vi "Find Pupil.vi"(11 "error in":errorcluster) -> (4 "Pupil Data":T1, 15 "error out":errorcluster)   [LabVIEW 2014]
uses:
  <vilib>/vision/NI_Vision_Development_Module.lvlib
panel:
  out "Image Out":T2(plugin-control)
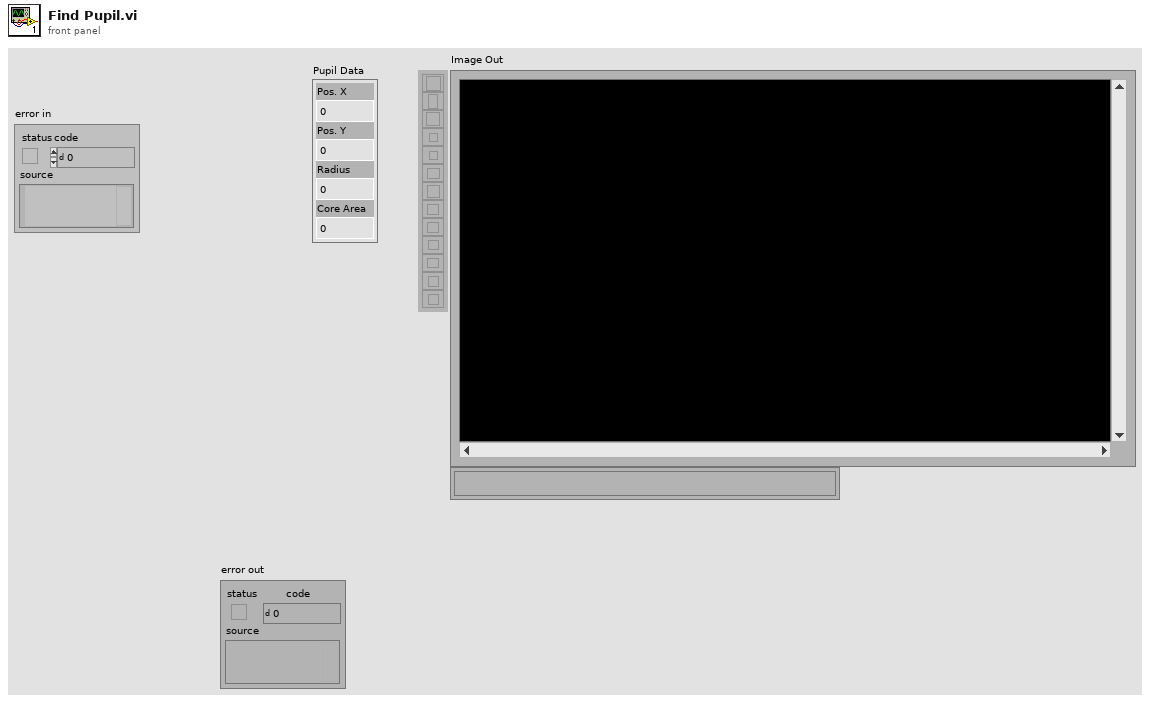
[diagram p1: front panel]
types:
  T1 = cluster{"Pos. X":i32, "Pos. Y":i32, "Radius":i32, "Core Area":i32}
  T2 = typedef "IMAQ Image.ctl" = refnum<image>
  T3 = cluster{"Left":i32, "Top":i32, "Right":i32, "Bottom":i32}
  T4 = typedef "Image Type" = u32
  T5 = cluster{"Pos. X":i32, "Pos. Y":i32, "Radius":i32, "Core Area":i32}[]
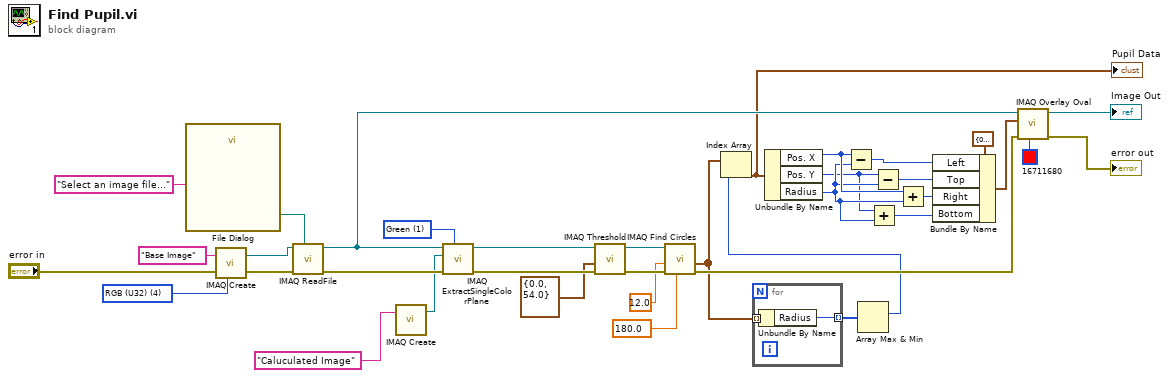
[diagram p0: block diagram]
diagram:
  w29 = 1 items=["Red", "Green", "Blue", "Hue", "Saturation", "Luminance", "Value", "Intensity"] ("Color Plane")
  w30 = T4 4 items=["Grayscale (U8)", "Grayscale (I16)", "Grayscale (SGL)", "Complex (CSG)", "RGB (U32)", "HSL (U32)", "RGB (U64)", "Grayscale (U16)"] ("Image Type")
  n1 = call "File Dialog"("prompt"="Select an image file...") -> ("selected path"=w31:path)  [unwired: 6 in, 8 out]
  n2 = call "IMAQ Create"("Image Name"="Base Image", "Image Type"=w30, "error in (no error)"="error in") -> ("New Image"=w35:T2, "error out"=w34:errorcluster)  [unwired: 1 in, 1 out]
  n3 = call "IMAQ ReadFile"("File Path"=w31, "error in (no error)"=w34, "Image"=w35) -> ("error out"=w36:errorcluster, "Image Out"=w19:T2)  [unwired: 2 in, 5 out]
  n4 = call "IMAQ Create"("Image Name"="Caluculated Image") -> ("New Image"=w20:T2)  [unwired: 3 in, 2 out]
  n5 = call "IMAQ ExtractSingleColorPlane"("Color Plane"=w29, "error in (no error)"=w36, "Image Dst"=w20, "Image Src"=w19) -> ("error out"=w28:errorcluster, "Image Dst Out"=w26:T2)  [unwired: 6 out]
  n6 = call "IMAQ Threshold"("error in (no error)"=w28, "Range"=cluster{"Lower value":sgl, "Upper value":sgl} {"Lower value"=0.0, "Upper value"=54.0}, "Image Src"=w26) -> ("error out"=w21:errorcluster, "Image Dst Out"=w24:T2)  [unwired: 3 in, 4 out]
  n7 = call "IMAQ Find Circles"("Max Radius"=sgl 180.0, "error in (no error)"=w21, "Min Radius"=sgl 12.0, "Image Src"=w24) -> ("error out"=w6:errorcluster, "Circles Data"=w4:T5)  [unwired: 1 in, 5 out]
  n8 = for {
    tunnel: w4 -> [w38] mode=indexing
    tunnel: [w37] -> w3 mode=indexing
    n9 = Unbundle By Name(w38) -> ("Radius"=w37:i32)
  }
  n10 = Array Max & Min(array=w3) -> (max index (indices)=w2:i32)  [unwired: 3 out]
  n11 = Index Array(array=w4, index=w2) -> (element=w17:T1)
  "Pupil Data" <- w17
  n12 = Unbundle By Name(w17) -> ("Pos. X"=w10:i32, "Pos. Y"=w7:i32, "Radius"=w9:i32)
  n13 = Subtract(x=w10, y=w9) -> (x-y=w13:i32)
  n14 = Add(x=w7, y=w9) -> (x+y=w8:i32)
  n15 = Subtract(x=w7, y=w9) -> (x-y=w12:i32)
  n16 = Add(x=w10, y=w9) -> (x+y=w11:i32)
  n17 = Bundle By Name(cluster=T3 {"Left"=0, "Top"=0, "Right"=0, "Bottom"=0} ("Bounding Rectangle"), "Left"=w13, "Top"=w12, "Right"=w11, "Bottom"=w8) -> (w14:T3)
  n18 = call "IMAQ Overlay Oval"("Color"=u32 16711680, "error in (no error)"=w6, "Bounding Rectangle"=w14, "Image"=w19) -> ("error out"=→"error out":errorcluster, "Image Out"=→"Image Out":T2)  [unwired: 6 in]
